vi "Export File - Tx Packet XML.vi"(4 "Tx Packet":T1 {"Endianness" items=["big-endian"=0, "little-endian"=2]}, 6 "RootNode":refnum<k24>, 8 "error in (no error)":errorcluster, 9 "Tx Packet Header Data":T5, 11 "XmlDocument in":refnum<k24>) -> (0 "error out":errorcluster, 3 "XmlDocument out":refnum<k24>)   [LabVIEW 2016, in "UDP-Custom-Device System Explorer.lvlib"]
uses:
  UDP-Custom-Device System Explorer.lvlib
  System.Xml
  Types/XML - New/ImpExp - Packet Headers.ctl
  Types/XML - New/ImpExp - Tx Packet Data.ctl
  <vilib>/NI Veristand/Custom Device API/Custom Device Item Info.ctl
  Shared/Types/Shared - Channel Data Type.ctl
  Shared/Types/Shared - Buffered.PacketInfo.ctl
  Shared/UDP-Custom-Device Shared.lvlib
  <vilib>/NI VeriStand/Custom Device API/Custom Device API.lvlib
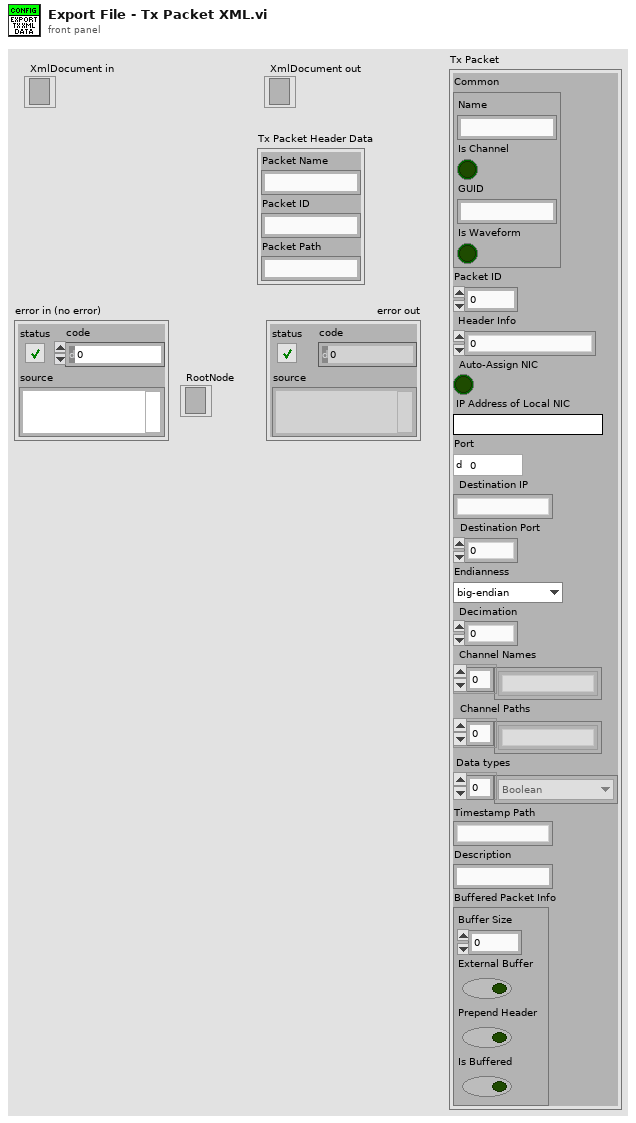
[diagram p1: front panel]
types:
  T1 = typedef "UDP-Custom-Device System Explorer.lvlib/ImpExp - Tx Packet Data.ctl" = cluster{"Common":T2, "Packet ID":i32, "Header Info":u32, "Auto-Assign NIC":bool, "IP Address of Local NIC":string, "Port":u16, "Destination IP":string, "Destination Port":u16, "Endianness":u16, "Decimation":u16, "Channel Names":string[], "Channel Paths":string[], "Data types":T3[], "Timestamp Path":string, "Description":string, "Buffered Packet Info":T4}
  T2 = typedef "Custom Device API.lvlib/Custom Device Item Info.ctl" = cluster{"Name":string, "Is Channel":bool, "GUID":string, "Is Waveform":bool}
  T3 = typedef "UDP-Custom-Device Shared.lvlib/Shared - Channel Data Type.ctl" = enum16{"Boolean", "Single", "Double", "I8", "I16", "I32", "I64", "U8", "U16", "U32", "U64"}
  T4 = typedef "UDP-Custom-Device Shared.lvlib/Shared - Buffered.PacketInfo.ctl" = cluster{"Buffer Size":i32, "External Buffer":bool, "Prepend Header":bool, "Is Buffered":bool}
  T5 = typedef "UDP-Custom-Device System Explorer.lvlib/ImpExp - Packet Headers.ctl" = cluster{"Packet Name":string, "Packet ID":string, "Packet Path":string}
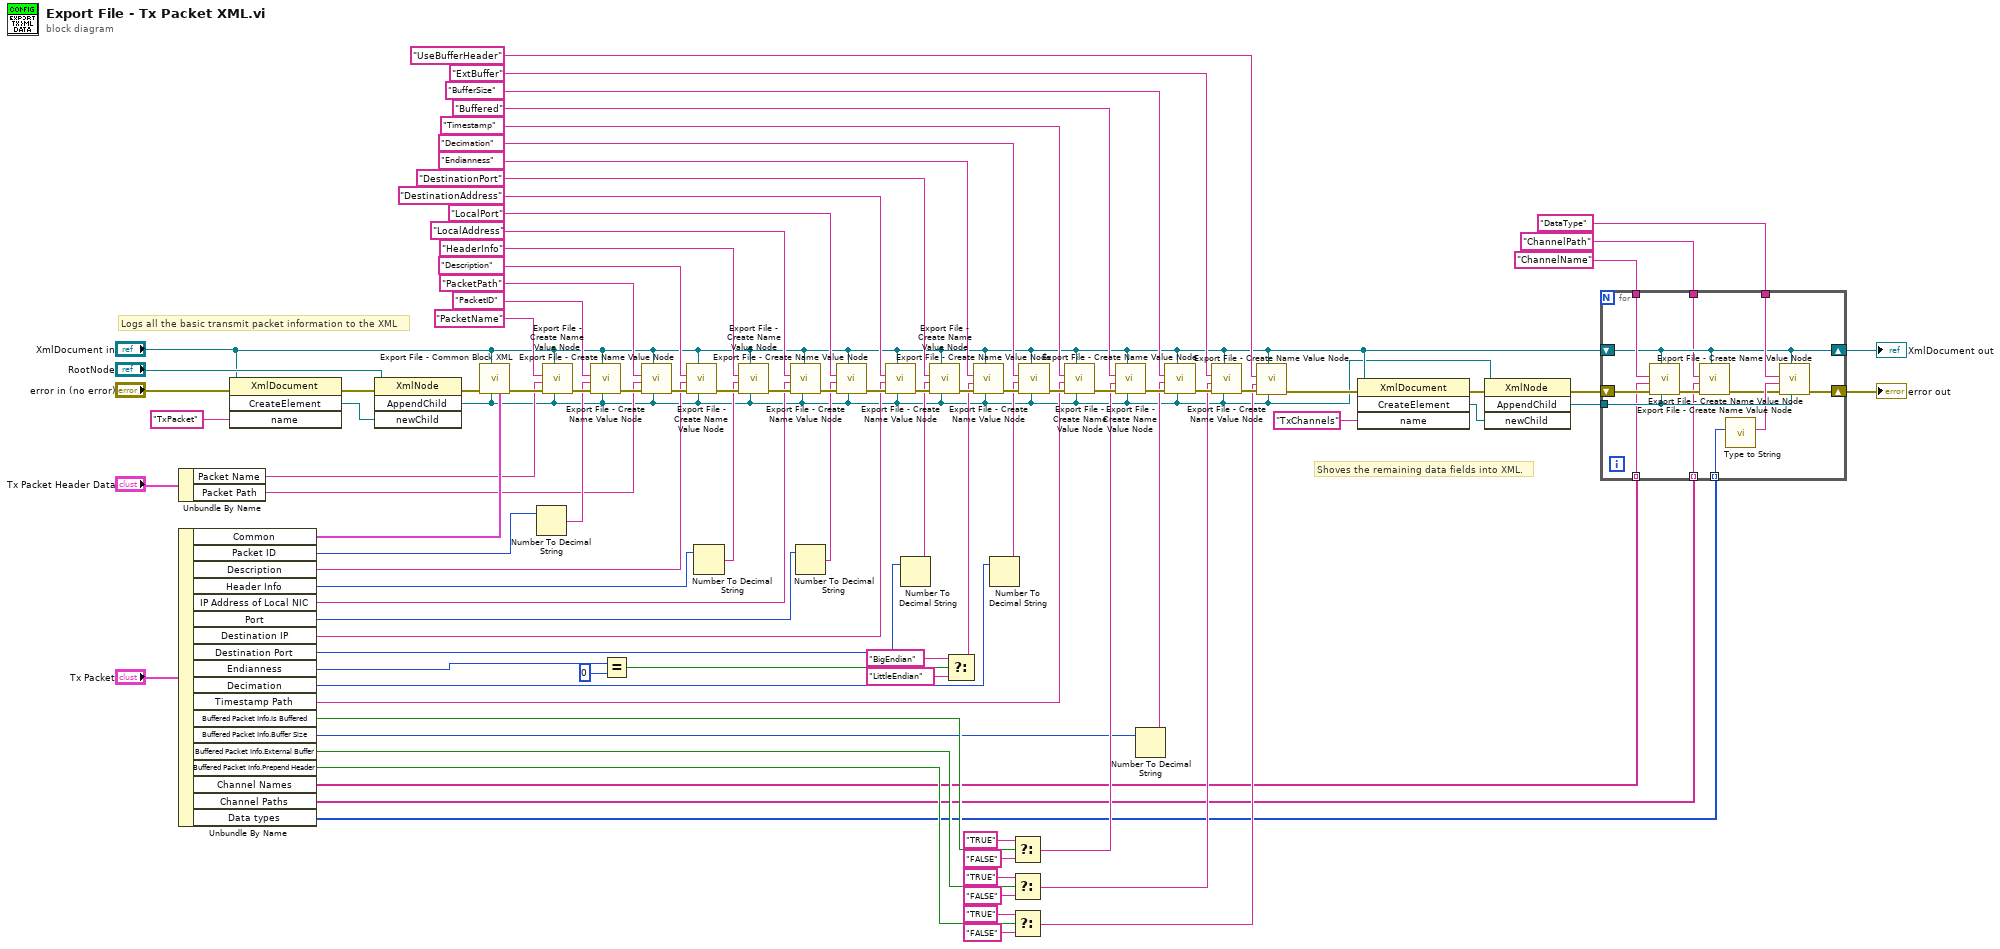
[diagram p0: block diagram]
diagram:
  # "Shoves the remaining data fields into XML."
  # "Logs all the basic transmit packet information to the XML"
  n1 = Unbundle By Name("Tx Packet Header Data") -> ("Packet Name"=w77:string, "Packet Path"=w75:string)
  n2 = Unbundle By Name("Tx Packet") -> ("Common"=w87:T2, "Packet ID"=w78:i32, "Description"=w52:string, "Header Info"=w51:u32, "IP Address of Local NIC"=w48:string, "Port"=w47:u16, "Destination IP"=w45:string, "Destination Port"=w44:u16, "Endianness"=w36:u16, "Decimation"=w42:u16, "Timestamp Path"=w40:string, "Buffered Packet Info.Is Buffered"=w31:bool, "Buffered Packet Info.Buffer Size"=w26:i32, "Buffered Packet Info.External Buffer"=w20:bool, "Buffered Packet Info.Prepend Header"=w19:bool, "Channel Names"=w4:string[], "Channel Paths"=w1:string[], "Data types"=w3:T3[])
  n3 = invoke class="XmlDocument" method="CreateElement"(reference="XmlDocument in", error in="error in (no error)", "name"="TxPacket" ("Tag Name")) -> (error out=w91:errorcluster, "CreateElement"=w92:refnum<k24>)  [unwired: 1 in, 2 out]
  n4 = invoke class="XmlNode" method="AppendChild"(reference="RootNode", error in=w91, "newChild"=w92) -> (error out=w90:errorcluster, "AppendChild"=w5:refnum<k24>)  [unwired: 1 in, 2 out]
  n5 = call "Export File - Common Block XML.vi"("Common"=w87, "RootNode in"=w5, "XmlDocument in"="XmlDocument in", "error in (no error)"=w90) -> ("error out"=w80:errorcluster)  [unwired: 7 in]
  n6 = Number To Decimal String(number=w78) -> (decimal integer string=w76:string)  [unwired: 1 in]
  n7 = call "Export File - Create Name Value Node.vi"("RootNode in"=w5, "XmlDocument in"="XmlDocument in", "error in (no error)"=w80, "Value"=w77, "Name"="PacketName" ("Tag Name")) -> ("error out"=w85:errorcluster)  [unwired: 6 in]
  n8 = call "Export File - Create Name Value Node.vi"("RootNode in"=w5, "XmlDocument in"="XmlDocument in", "error in (no error)"=w85, "Value"=w76, "Name"="PacketID" ("Tag Name")) -> ("error out"=w84:errorcluster)  [unwired: 6 in]
  n9 = Equal?(x=w36, y=u16 0) -> (x = y?=w35:bool)
  n10 = call "Export File - Create Name Value Node.vi"("RootNode in"=w5, "XmlDocument in"="XmlDocument in", "error in (no error)"=w84, "Value"=w75, "Name"="PacketPath" ("Tag Name")) -> ("error out"=w67:errorcluster)  [unwired: 6 in]
  n11 = call "Export File - Create Name Value Node.vi"("RootNode in"=w5, "XmlDocument in"="XmlDocument in", "error in (no error)"=w67, "Value"=w52, "Name"="Description" ("Tag Name")) -> ("error out"=w74:errorcluster)  [unwired: 6 in]
  n12 = Number To Decimal String(number=w51) -> (decimal integer string=w50:string)  [unwired: 1 in]
  n13 = call "Export File - Create Name Value Node.vi"("RootNode in"=w5, "XmlDocument in"="XmlDocument in", "error in (no error)"=w74, "Value"=w50, "Name"="HeaderInfo" ("Tag Name")) -> ("error out"=w49:errorcluster)  [unwired: 6 in]
  n14 = call "Export File - Create Name Value Node.vi"("RootNode in"=w5, "XmlDocument in"="XmlDocument in", "error in (no error)"=w49, "Value"=w48, "Name"="LocalAddress" ("Tag Name")) -> ("error out"=w73:errorcluster)  [unwired: 6 in]
  n15 = Number To Decimal String(number=w47) -> (decimal integer string=w46:string)  [unwired: 1 in]
  n16 = call "Export File - Create Name Value Node.vi"("RootNode in"=w5, "XmlDocument in"="XmlDocument in", "error in (no error)"=w73, "Value"=w46, "Name"="LocalPort" ("Tag Name")) -> ("error out"=w72:errorcluster)  [unwired: 6 in]
  n17 = call "Export File - Create Name Value Node.vi"("RootNode in"=w5, "XmlDocument in"="XmlDocument in", "error in (no error)"=w72, "Value"=w45, "Name"="DestinationAddress" ("Tag Name")) -> ("error out"=w71:errorcluster)  [unwired: 6 in]
  n18 = Number To Decimal String(number=w44) -> (decimal integer string=w43:string)  [unwired: 1 in]
  n19 = call "Export File - Create Name Value Node.vi"("RootNode in"=w5, "XmlDocument in"="XmlDocument in", "error in (no error)"=w71, "Value"=w43, "Name"="DestinationPort" ("Tag Name")) -> ("error out"=w70:errorcluster)  [unwired: 6 in]
  n20 = Select(t="BigEndian", s=w35, f="LittleEndian") -> (s? t:f=w34:string)
  n21 = call "Export File - Create Name Value Node.vi"("RootNode in"=w5, "XmlDocument in"="XmlDocument in", "error in (no error)"=w70, "Value"=w34, "Name"="Endianness" ("Tag Name")) -> ("error out"=w69:errorcluster)  [unwired: 6 in]
  n22 = Number To Decimal String(number=w42) -> (decimal integer string=w41:string)  [unwired: 1 in]
  n23 = Select(t="TRUE", s=w31, f="FALSE") -> (s? t:f=w28:string)
  n24 = Select(t="TRUE", s=w20, f="FALSE") -> (s? t:f=w18:string)
  n25 = Select(t="TRUE", s=w19, f="FALSE") -> (s? t:f=w17:string)
  n26 = call "Export File - Create Name Value Node.vi"("RootNode in"=w5, "XmlDocument in"="XmlDocument in", "error in (no error)"=w69, "Value"=w41, "Name"="Decimation" ("Tag Name")) -> ("error out"=w68:errorcluster)  [unwired: 6 in]
  n27 = call "Export File - Create Name Value Node.vi"("RootNode in"=w5, "XmlDocument in"="XmlDocument in", "error in (no error)"=w68, "Value"=w40, "Name"="Timestamp" ("Tag Name")) -> ("error out"=w30:errorcluster)  [unwired: 6 in]
  n28 = call "Export File - Create Name Value Node.vi"("RootNode in"=w5, "XmlDocument in"="XmlDocument in", "error in (no error)"=w30, "Value"=w28, "Name"="Buffered" ("Tag Name")) -> ("error out"=w29:errorcluster)  [unwired: 6 in]
  n29 = Number To Decimal String(number=w26) -> (decimal integer string=w25:string)  [unwired: 1 in]
  n30 = call "Export File - Create Name Value Node.vi"("RootNode in"=w5, "XmlDocument in"="XmlDocument in", "error in (no error)"=w29, "Value"=w25, "Name"="BufferSize" ("Tag Name")) -> ("error out"=w56:errorcluster)  [unwired: 6 in]
  n31 = call "Export File - Create Name Value Node.vi"("RootNode in"=w5, "XmlDocument in"="XmlDocument in", "error in (no error)"=w56, "Value"=w18, "Name"="ExtBuffer" ("Tag Name")) -> ("error out"=w55:errorcluster)  [unwired: 6 in]
  n32 = call "Export File - Create Name Value Node.vi"("RootNode in"=w5, "XmlDocument in"="XmlDocument in", "error in (no error)"=w55, "Value"=w17, "Name"="UseBufferHeader" ("Tag Name")) -> ("error out"=w9:errorcluster)  [unwired: 6 in]
  n33 = invoke class="XmlDocument" method="CreateElement"(reference="XmlDocument in", error in=w9, "name"="TxChannels" ("Tag Name")) -> (error out=w14:errorcluster, "CreateElement"=w16:refnum<k24>)  [unwired: 1 in, 2 out]
  n34 = invoke class="XmlNode" method="AppendChild"(reference=w5, error in=w14, "newChild"=w16) -> (error out=w13:errorcluster, "AppendChild"=w12:refnum<k24>)  [unwired: 1 in, 2 out]
  n35 = for {
    shift-right: [w105] -> w8
    shift-left: w13 -> [w106]
    tunnel: w12 -> [w104]
    shift-right: [w98] -> w6
    shift-left: "XmlDocument in" -> [w98]
    tunnel: "ChannelName" ("Tag Name") -> [w103]
    tunnel: "DataType" ("Tag Name") -> [w102]
    tunnel: w4 -> [w101] mode=indexing
    tunnel: w3 -> [w100] mode=indexing
    tunnel: "ChannelPath" ("Tag Name") -> [w95]
    tunnel: w1 -> [w94] mode=indexing
    n36 = call "Export File - Create Name Value Node.vi"("RootNode in"=w104, "XmlDocument in"=w98, "error in (no error)"=w106, "Value"=w101, "Name"=w103) -> ("error out"=w97:errorcluster)  [unwired: 6 in]
    n37 = call "Export File - Create Name Value Node.vi"("XmlDocument in"=w98, "error in (no error)"=w97, "Value"=w94, "Name"=w95) -> ("error out"=w96:errorcluster)  [unwired: 7 in]
    n38 = call "Type to String.vi"("Data Type"=w100) -> ("String Type"=w99:string)  [unwired: 10 in]
    n39 = call "Export File - Create Name Value Node.vi"("RootNode in"=w104, "XmlDocument in"=w98, "error in (no error)"=w96, "Value"=w99, "Name"=w102) -> ("error out"=w105:errorcluster)  [unwired: 6 in]
  }
  "error out" <- w8
  "XmlDocument out" <- w6
